vi "convert_binData_to_integerArray.vi"(3 "Bin Number Integer Format":T1, 5 "Bin Data":string) -> (0 "Array size":i32, 1 "Numbers out":i32[](array[numeric]), 2 "Bin Data Aligned":bool)   [LabVIEW 2022 SP3, in "hmp4000_rsidr_core.lvlib"]
uses:
  hmp4000_rsidr_core.lvlib
  type_Binary_Integer_Number_Format.ctl
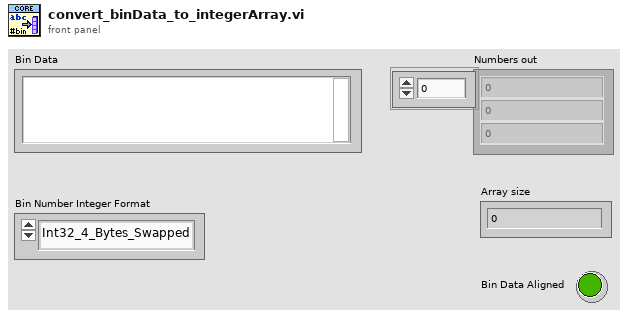
[diagram p1: front panel]
types:
  T1 = typedef "hmp4000_rsidr_core.lvlib/type_Binary_Integer_Number_Format.ctl" = enum16{"Int32_4_Bytes_Swapped", "Int32_4 Bytes", "Int16_2_Bytes_Swapped", "Int16_2_Bytes"}
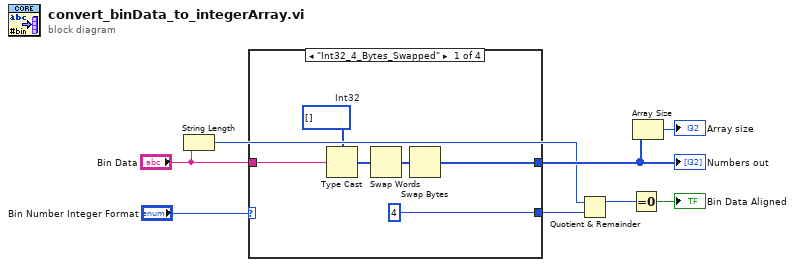
[diagram p0: block diagram]
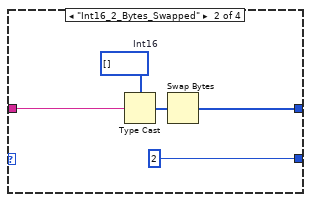
[diagram p2: hidden frame]
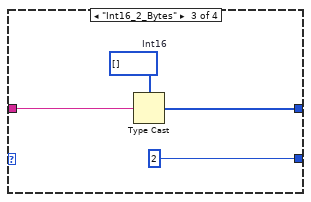
[diagram p3: hidden frame]
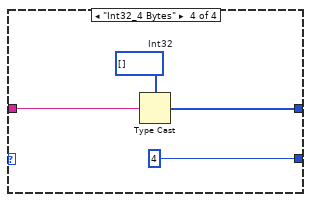
[diagram p4: hidden frame]
diagram:
  n1 = String Length(string="Bin Data") -> (length=w2:i32)
  n2 = case shown="\"Int32_4_Bytes_Swapped\"" "Bin Number Integer Format" {
    tunnel: [w10 w17 w21 w26] -> w7
    tunnel: "Bin Data" -> [w11 w18 w22 w25]
    tunnel: [4 ("y") 2 ("y") 2 ("y") 4 ("y")] -> w1
    frame "Int32_4_Bytes_Swapped" {
      w12 = i32[] []  # Int32
      n3 = Type Cast(type=w12, x=w11) -> (*(type *) &x=w14:i32[])
      n4 = Swap Words(1:w14) -> (0:w13:i32[])
      n5 = Swap Bytes(anything=w13) -> (byte swapped=w10:i32[])
    }
    frame "Int16_2_Bytes_Swapped" {
      w19 = i16[] []  # Int16
      n6 = Type Cast(type=w19, x=w18) -> (*(type *) &x=w16:i16[])
      n7 = Swap Bytes(anything=w16) -> (byte swapped=w17:i16[])
    }
    frame "Int16_2_Bytes" {
      w23 = i16[] []  # Int16
      n8 = Type Cast(type=w23, x=w22) -> (*(type *) &x=w21:i16[])
    }
    frame "Int32_4 Bytes" {
      w27 = i32[] []  # Int32
      n9 = Type Cast(type=w27, x=w25) -> (*(type *) &x=w26:i32[])
    }
  }
  "Numbers out" <- w7
  n10 = Quotient & Remainder(x=w2, y=w1) -> (x-y*floor(x/y)=w4:i32)  [unwired: 1 out]
  n11 = Equal To 0?(x=w4) -> (x = 0?=→"Bin Data Aligned":bool)
  n12 = Array Size(array=w7) -> (size(s)=→"Array size":i32)
